vi "ShooterMotorAndEncoderTest.vi"(9 "Progress":string, 11 "ProgressText":string) -> (1 "EndTestText":string)   [LabVIEW 2012]
panel:
  in  "EncoderGuide":dbl=3000.0
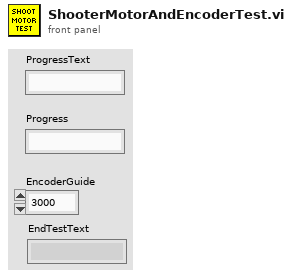
[diagram p1: front panel]
types:
  T1 = typedef "WPI_MotorControlDeviceRef.ctl" = cluster{"DeviceStatus":errorcluster, "Type":enum16{"PWM", "CAN"}, "PWM":cluster{"Digital Module":T2, "PWM Channel":T3, "DeadBand":T4}, "CAN":cluster{"Device Number":u8, "Control Mode":T5, "Semaphore":T6, "Max Vout":dbl}, "Invert":bool, "TransformRef":T7, "InvTransformRef":T7}
  T2 = typedef "FPGA_TypedefDigitalModule.ctl" = enum16{"Digital Module 1", "Digital Module 2"}
  T3 = typedef "FPGA_DIOPWMChannel.ctl" = enum8{"PWM 1", "PWM 2", "PWM 3", "PWM 4", "PWM 5", "PWM 6", "PWM 7", "PWM 8", "PWM 9", "PWM 10", "Invalid"}
  T4 = typedef "WPI_PWMDeadband.ctl" = cluster{"Name":string, "maxPositivePwm":i32, "minPositivePwm":i32, "centerPwm":i32, "maxNegativePwm":i32, "minNegativePwm":i32, "angularRange":u16}
  T5 = typedef "WPI_CANJaguar_ControlMode.ctl" = enum8{"Percent VBus", "Current", "Speed", "Position", "Voltage"}
  T6 = typedef "Semaphore RefNum" = refnum<k1>
  T7 = typedef "WPI_PWMTransform_ConPane.ctl" = refnum<vi>
  T8 = typedef "WPI_EncoderDevRef.ctl" = cluster{"DevStatus":errorcluster, "EncoderIndex":T9, "CounterIndex":T10, "DistancePerCount":dbl, "Decoding Type":T11}
  T9 = typedef "FPGA_EncoderIdx.ctl" = enum8{"Enc 0", "Enc 1", "Enc 2", "Enc 3", "Invalid"}
  T10 = typedef "FPGA_CounterCtrSystemIndex.ctl" = enum8{"Ctr 0", "Ctr 1", "Ctr 2", "Ctr 3", "Ctr 4", "Ctr 5", "Ctr 6", "Ctr 7", "Invalid"}
  T11 = typedef "WPI_EncoderType.ctl" = enum16{"1x", "2x", "4x"}
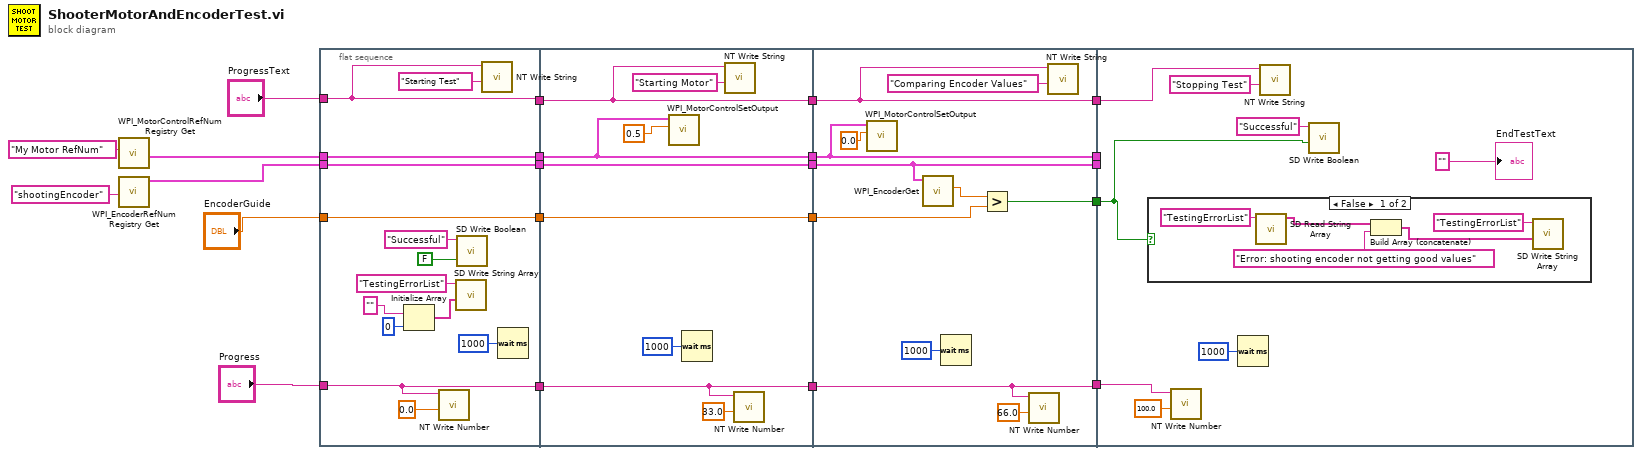
[diagram p0: block diagram]
diagram:
  n1 = call <vilib>:"WPI_MotorControlRefNum Registry Get.vi"("refnum name"="My Motor RefNum") -> ("MotorControlDevRef"=w5:T1)  [unwired: 9 in, 1 out]
  n2 = call <vilib>:"WPI_EncoderRefNum Registry Get.vi"("refnum name"="shootingEncoder") -> ("EncoderDevRef"=w4:T8)  [unwired: 9 in, 1 out]
  n3 = flat-sequence {
    tunnel: "ProgressText" -> [w35]
    tunnel: "Progress" -> [w34]
    tunnel: [w35] -> w22
    tunnel: [w34] -> w21
    tunnel: [w31] -> w20
    tunnel: w5 -> [w31]
    tunnel: [w30] -> w19
    tunnel: w4 -> [w30]
    tunnel: "EncoderGuide" -> [w27]
    tunnel: [w27] -> w18
    tunnel: w22 -> [w40]
    tunnel: w21 -> [w38]
    tunnel: w20 -> [w42]
    tunnel: w19 -> [w45]
    tunnel: [w40] -> w17
    tunnel: [w38] -> w16
    tunnel: [w45] -> w15
    tunnel: [w42] -> w14
    tunnel: [w39] -> w13
    tunnel: w18 -> [w39]
    tunnel: w17 -> [w48]
    tunnel: w16 -> [w47]
    tunnel: w15 -> [w54]
    tunnel: w14 -> [w55]
    tunnel: w13 -> [w52]
    tunnel: [w48] -> w12
    tunnel: [w47] -> w11
    tunnel: [w54] -> w10
    tunnel: [w55] -> w9
    tunnel: [w51] -> w8
    tunnel: w12 -> [w61]
    tunnel: w11 -> [w60]
    tunnel: w10 -> [_]
    tunnel: w9 -> [_]
    tunnel: w8 -> [w57]
    frame #0 {
      n4 = Initialize Array("", 0 ("dimension size")) -> (w24:string[])
      n5 = call <vilib>:"NT Write Number.vi"("Numeric"=0.0, "Name"=w34) -> ()  [unwired: 9 in, 1 out]
      n6 = call <vilib>:"SD Write String Array.vi"("String Array"=w24, "Name"="TestingErrorList") -> ()  [unwired: 8 in, 2 out]
      n7 = call <vilib>:"SD Write Boolean.vi"("Boolean"=FALSE, "Name"="Successful") -> ()  [unwired: 8 in, 2 out]
      n8 = call <vilib>:"NT Write String.vi"("String"="Starting Test", "Name"=w35) -> ()  [unwired: 9 in, 1 out]
      n9 = Wait (ms)(milliseconds to wait=u32 1000) -> ()  [unwired: 1 out]
    }
    frame #1 {
      n10 = call <vilib>:"WPI_MotorControlSetOutput.vi"("Output"=0.5, "MotorControlDevRef"=w42) -> ()  [unwired: 7 in, 3 out]
      n11 = Wait (ms)(milliseconds to wait=u32 1000) -> ()  [unwired: 1 out]
      n12 = call <vilib>:"NT Write String.vi"("String"="Starting Motor", "Name"=w40) -> ()  [unwired: 9 in, 1 out]
      n13 = call <vilib>:"NT Write Number.vi"("Numeric"=33.0, "Name"=w38) -> ()  [unwired: 9 in, 1 out]
    }
    frame #2 {
      n14 = call <vilib>:"WPI_MotorControlSetOutput.vi"("Output"=0.0, "MotorControlDevRef"=w55) -> ()  [unwired: 7 in, 3 out]
      n15 = call <vilib>:"WPI_EncoderGet.vi"("EncoderDevRef"=w54) -> ("Distance"=w53:dbl)  [unwired: 5 in, 5 out]
      n16 = Wait (ms)(milliseconds to wait=u32 1000) -> ()  [unwired: 1 out]
      n17 = Greater?(x=w53, y=w52) -> (0:w51:bool)
      n18 = call <vilib>:"NT Write Number.vi"("Numeric"=66.0, "Name"=w47) -> ()  [unwired: 9 in, 1 out]
      n19 = call <vilib>:"NT Write String.vi"("String"="Comparing Encoder Values", "Name"=w48) -> ()  [unwired: 9 in, 1 out]
    }
    frame #3 {
      n20 = case shown="False" w57 {
        frame False {
          n21 = call <vilib>:"SD Read String Array.vi"("Name"="TestingErrorList") -> ("String Array"=w65:string[])  [unwired: 9 in, 1 out]
          n22 = Build Array (concatenate)(w65, "Error: shooting encoder not getting good values" ("String")) -> (w67:string[])
          n23 = call <vilib>:"SD Write String Array.vi"("String Array"=w67, "Name"="TestingErrorList") -> ()  [unwired: 8 in, 2 out]
        }
        frame True {
        }
      }
      n24 = call <vilib>:"NT Write Number.vi"("Numeric"=100.0, "Name"=w60) -> ()  [unwired: 9 in, 1 out]
      n25 = Wait (ms)(milliseconds to wait=u32 1000) -> ()  [unwired: 1 out]
      n26 = call <vilib>:"NT Write String.vi"("String"="Stopping Test", "Name"=w61) -> ()  [unwired: 9 in, 1 out]
      n27 = call <vilib>:"SD Write Boolean.vi"("Boolean"=w57, "Name"="Successful") -> ()  [unwired: 8 in, 2 out]
      "EndTestText" <- "" ("EndTestText")
    }
  }
